vi "Set Custom Device Instance Name.vi"(8 "error in":errorcluster, 11 "Item Ref in":u64 format="%.0x") -> (0 "error out":errorcluster, 3 "Item Ref out":u64 format="%.0x")   [LabVIEW 2026]
uses:
  NationalInstruments.VeriStand.SystemDefinitionAPI
  Template Configuration.lvlib
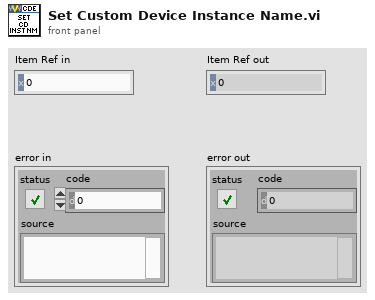
[diagram p1: front panel]
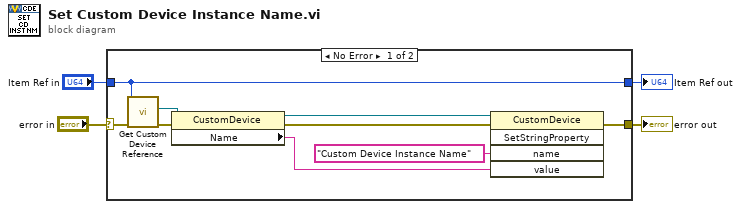
[diagram p0: block diagram]
diagram:
  n1 = case shown="No Error" "error in" {
    selector: "error in" -> [w5 w15]
    tunnel: [w12 w15] -> w3
    tunnel: "Item Ref in" -> [w6 w14]
    tunnel: [w6 w14] -> w1
    frame No Error {
      n2 = call "Get Custom Device Reference.vi"("error in"=w5, "Item Ref in"=w6) -> ("error out"=w7:errorcluster, "Custom Device"=w8:refnum<k24>)  [unwired: 7 in, 1 out]
      n3 = property class="CustomDevice"(reference=w8, error in=w7) -> (reference out=w11:refnum<k24>, error out=w13:errorcluster, "Name"=w10:string)
      n4 = invoke class="CustomDevice" method="SetStringProperty"(reference=w11, error in=w13, "name"="Custom Device Instance Name", "value"=w10) -> (error out=w12:errorcluster)  [unwired: 1 in, 4 out]
    }
    frame Error {
    }
  }
  "error out" <- w3
  "Item Ref out" <- w1
